vi "TDMS Save Mode (SubVI).vi"(8 "error in (no error)":errorcluster, 11 "Raw Data Mode":string) -> ()   [LabVIEW 2019]
doc: "Based on configuration settings, this VI asserts the save interval for the 3 phase raw data. \n\nSince the 3ph Power process can be configured to capture data up to 50 kHz, this can result in a large volume of data. MODAQ provides three save modes for this data:\n1. Continuous (all data saved) \n2. None (no data saved)\n3. Interval\n\nInterval data saving allows for the user to record X minutes of data every Y minutes. For instance: 15 minutes of data every 60 minutes or 1 minute of data ever 5 minutes. X and Y can be any number of minutes as long as Y > X. These values are set in the Configurator app and loaded when MODAQ starts.\n\n2020 NREL"
uses:
  Globals and Definitions/Initialization Globals.vi
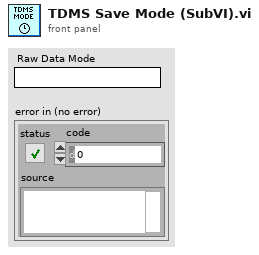
[diagram p1: front panel]
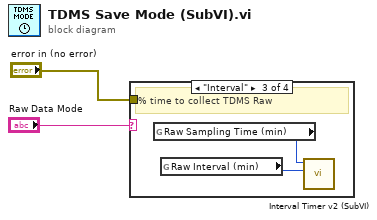
[diagram p0: block diagram]
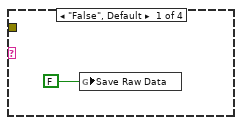
[diagram p2: hidden frame]
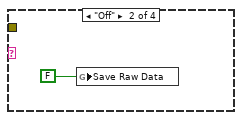
[diagram p3: hidden frame]
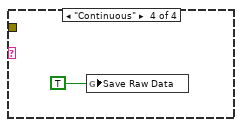
[diagram p4: hidden frame]
diagram:
  n1 = case shown="\"Interval\"" "Raw Data Mode" {
    tunnel: "error in (no error)" -> [_ _ _ _]
    frame "False", Default {
      n2 = global write "Initialization Globals.vi" "Save Raw Data"(FALSE ("Pow Interval Timer")) -> ()
    }
    frame "Off" {
      n3 = global write "Initialization Globals.vi" "Save Raw Data"(FALSE ("Pow Interval Timer")) -> ()
    }
    frame "Interval" {
      # "% time to collect TDMS Raw"
      n4 = global read "Initialization Globals.vi" "Raw Sampling Time (min)"() -> (w5:i32)
      n5 = global read "Initialization Globals.vi" "Raw Interval (min)"() -> (w6:i32)
      n6 = call "Interval Timer v2 (SubVI).vi"("Interval Time"=w6, "Sampling Time"=w5) -> ()  [unwired: 10 in]
    }
    frame "Continuous" {
      n7 = global write "Initialization Globals.vi" "Save Raw Data"(TRUE ("Pow Interval Timer")) -> ()
    }
  }
